vi "init_hw.vi"(8 "error in (no error)":errorcluster, 11 "dummyStageRapid in":refnum<class "dummyStageRapid.lvclass">) -> (0 "error out":errorcluster, 2 "Boolean":bool=TRUE, 3 "dummyStageRapid out":refnum<class "dummyStageRapid.lvclass">)   [LabVIEW 2019, in "dummyStageRapid.lvlib" / "dummyStageRapid.lvclass"]
uses:
  dummyStageRapid.lvclass
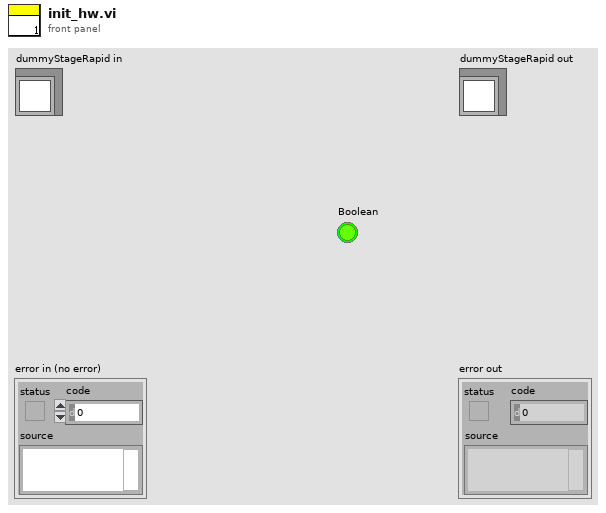
[diagram p1: front panel]
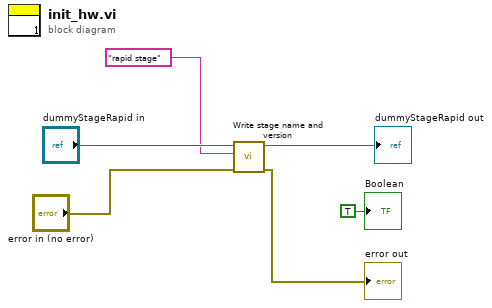
[diagram p0: block diagram]
diagram:
  n1 = call-dynamic "Write stage name and version.vi"("error in (no error)"="error in (no error)", "stage name and version"="rapid stage", "_stage in"="dummyStageRapid in") -> ("error out"=→"error out":errorcluster, "_stage out"=→"dummyStageRapid out":refnum<class "dummyStageRapid.lvclass">)  [unwired: 7 in]
  "Boolean" <- TRUE ("Boolean")
